vi "找球.vi"(1 "抬球电机继电器":T1, 2 "错误输入":errorcluster, 3 "光电门":T1, 4 "I/O":T11) -> (0 "错误输出":errorcluster)   [LabVIEW 2016]
uses:
  <vilib>/myRIO/Instrument Drivers/Onboard IO/PWM/typedefs/PWM Reference.ctl
  <vilib>/myRIO/Common/Instrument Driver Framework/Utilities/typedefs/myRIO Generic Hardware Reference.ctl
  <vilib>/myRIO/Common/Instrument Driver Framework/Utilities/typedefs/Hardware Version Enum.ctl
  <vilib>/myRIO/Common/Instrument Driver Framework/Utilities/typedefs/myRIO v1.0 Reference.ctl
  <vilib>/myRIO/Common/Instrument Driver Framework/Utilities/typedefs/Generic FPGA Reference.ctl
  <vilib>/myRIO/Common/Instrument Driver Framework/myRIO v1.0/PWM/typedefs/PWM Channels Enum.ctl
  <vilib>/myRIO/Instrument Drivers/Onboard IO/PWM/typedefs/PWM Configuration.ctl
  <vilib>/myRIO/Instrument Drivers/Onboard IO/DIO/typedefs/DIO Reference.ctl
  <vilib>/myRIO/Common/Instrument Driver Framework/myRIO v1.0/DIO/typedefs/DIO Channels List.ctl
  <vilib>/myRIO/Common/Instrument Driver Framework/myRIO v1.0/DIO/typedefs/DIO Channels Enum.ctl
  <vilib>/Utility/error.llb/Error Cluster From Error Code.vi
  <vilib>/myRIO/Common/Instrument Driver Framework/myRIO v1.0/DIO/vis/myRIO v1.0 Read DIO.vi
  <vilib>/myRIO/Common/Instrument Driver Framework/myRIO v1.0/DIO/vis/myRIO v1.0 Write DIO.vi
  <vilib>/myRIO/Instrument Drivers/Onboard IO/DIO/DIO.lvlib
  <vilib>/myRIO/Instrument Drivers/Onboard IO/PWM/PWM.lvlib
panel:
  out "error out":errorcluster
  out "拟合结果":T12
  out "速度":dbl[](array[numeric])
  out "前进一":bool
  out "前进二":bool
  out "旋转二":bool
  out "旋转一":bool
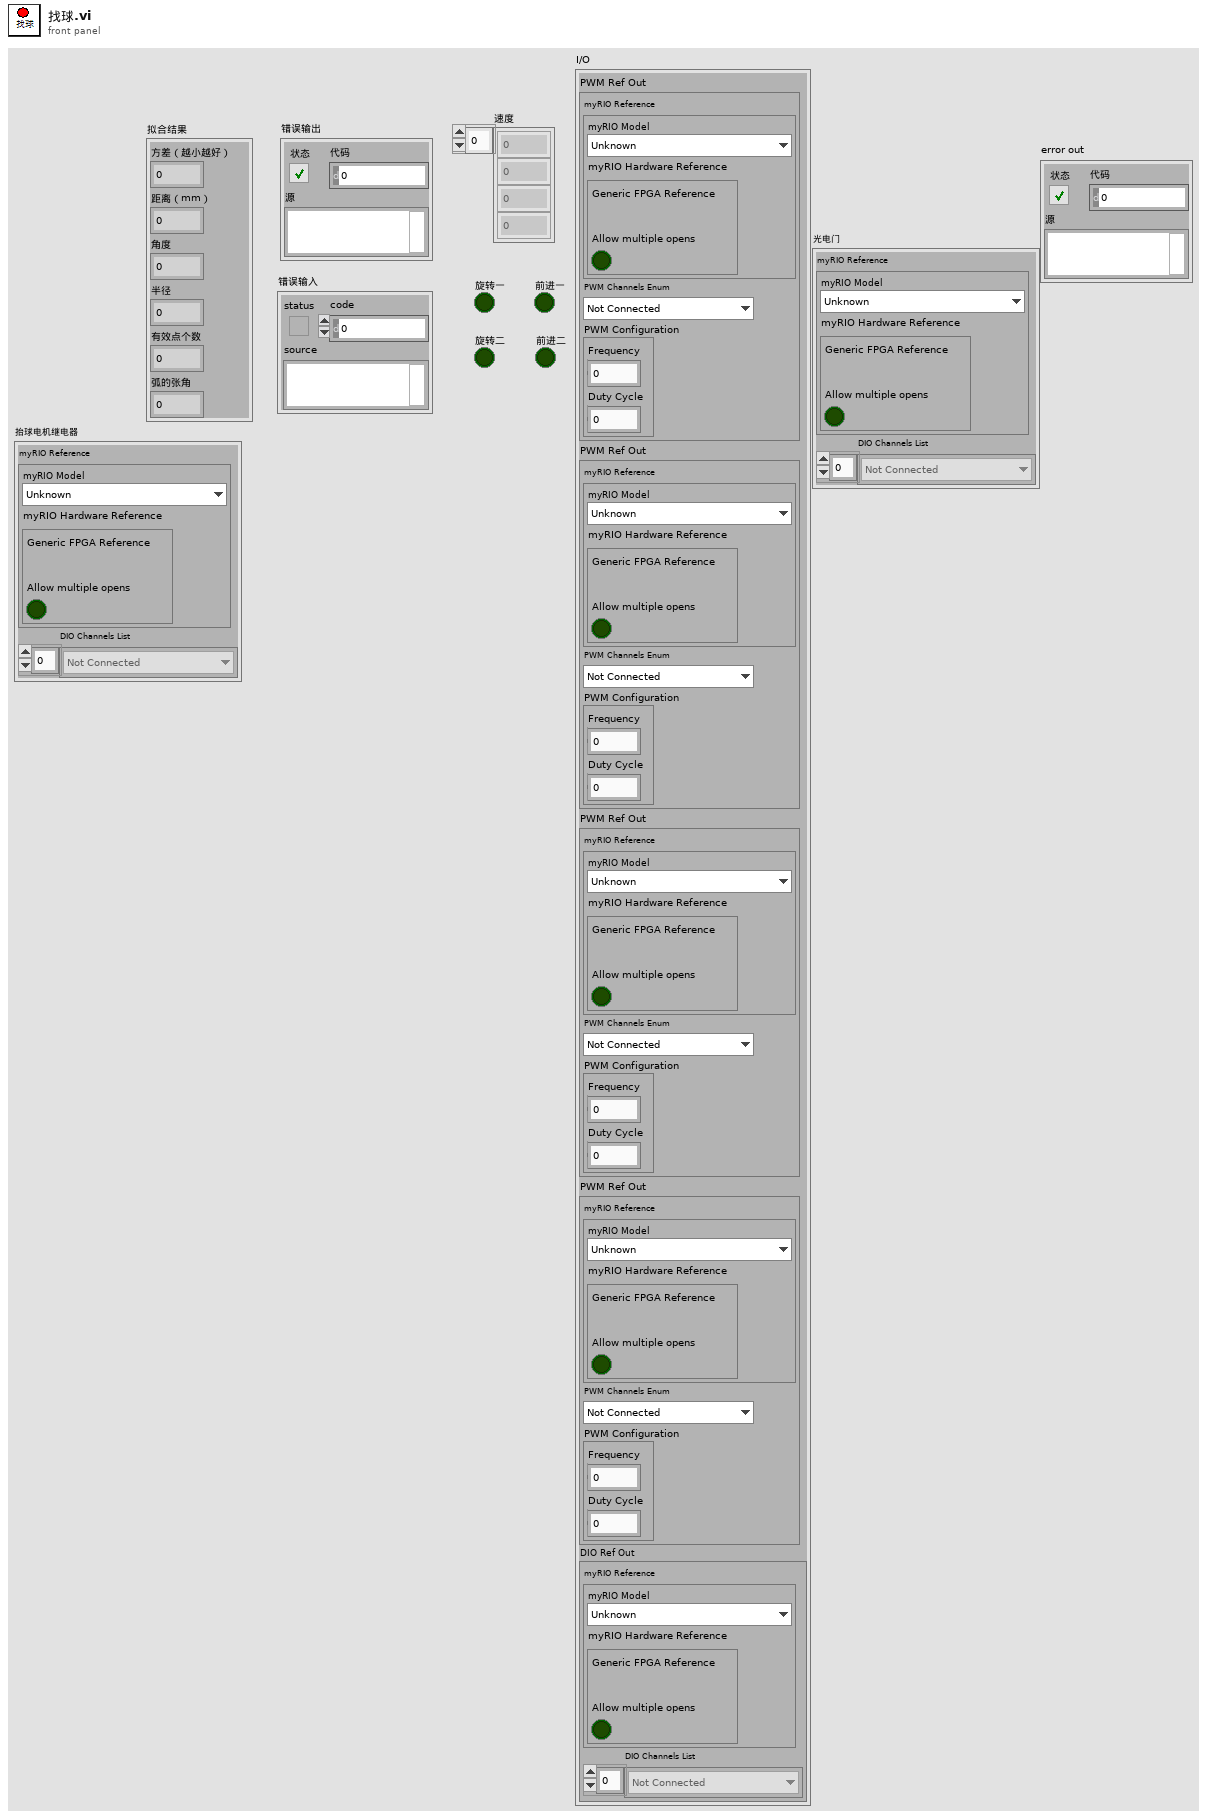
[diagram p1: front panel]
types:
  T1 = typedef "DIO.lvlib/DIO Reference.ctl" = cluster{"myRIO Reference":T2, "DIO Channels List":T6}
  T2 = typedef "myRIO Generic Hardware Reference.ctl" = cluster{"myRIO Model":T3, "myRIO Hardware Reference":T4}
  T3 = typedef "Hardware Version Enum.ctl" = enum16{"Unknown", "myRIO-1900", "myRIO-1950", "roboRIO", "NI ELVIS RIO CM"}
  T4 = typedef "myRIO v1.0 Reference.ctl" = cluster{"Generic FPGA Reference":T5, "Allow multiple opens":bool}
  T5 = typedef "Generic FPGA Reference.ctl" = refnum<k20>
  T6 = typedef "DIO Channels List.ctl" = T7[]
  T7 = typedef "DIO Channels Enum.ctl" = enum16{"Not Connected", "C/DIO0", "C/DIO1", "C/DIO2", "C/DIO3", "C/DIO4", "C/DIO5", "C/DIO6", "C/DIO7", "A/DIO0", "A/DIO1", "A/DIO2", "A/DIO3", "A/DIO4", "A/DIO5", "A/DIO6", "A/DIO7", "A/DIO8", "A/DIO9", "A/DIO10", "A/DIO11", "A/DIO12", "A/DIO13", "A/DIO14", "A/DIO15", "B/DIO0", "B/DIO1", "B/DIO2", "B/DIO3", "B/DIO4", "B/DIO5", "B/DIO6", "B/DIO7", "B/DIO8", "B/DIO9", "B/DIO10", "B/DIO11", "B/DIO12", "B/DIO13", "B/DIO14", "B/DIO15", "LED0", "LED1", "LED2", "LED3", "Button0", "DIO/DIO0", "DIO/DIO1", "DIO/DIO2", "DIO/DIO3", "DIO/DIO4", "DIO/DIO5", "DIO/DIO6", "DIO/DIO7", "DIO/DIO8", "DIO/DIO9", "SPI/CS0", "SPI/CS1", "SPI/CS2", "SPI/CS3", "LED RADIO (Green)", "LED RADIO (Red)", "LED COMM (Green)", "LED COMM (Red)", "LED MODE (Green)", "LED MODE (Red)"}
  T8 = typedef "PWM.lvlib/PWM Reference.ctl" = cluster{"myRIO Reference":T2, "PWM Channels Enum":T9, "PWM Configuration":T10}
  T9 = typedef "PWM Channels Enum.ctl" = enum16{"Not Connected", "C/PWM0", "C/PWM1", "A/PWM0", "A/PWM1", "A/PWM2", "B/PWM0", "B/PWM1", "B/PWM2", "PWM/PWM0", "PWM/PWM1", "PWM/PWM2", "PWM/PWM3", "PWM/PWM4", "PWM/PWM5", "PWM/PWM6", "PWM/PWM7", "PWM/PWM8", "PWM/PWM9"}
  T10 = typedef "PWM.lvlib/PWM Configuration.ctl" = cluster{"Frequency":dbl, "Duty Cycle":dbl}
  T11 = cluster{"PWM Ref Out":T8, "PWM Ref Out":T8, "PWM Ref Out":T8, "PWM Ref Out":T8, "DIO Ref Out":T1}
  T12 = cluster{"方差（越小越好）":dbl, "距离（mm）":dbl, "角度":dbl, "半径":dbl, "有效点个数":i32, "弧的张角":dbl}
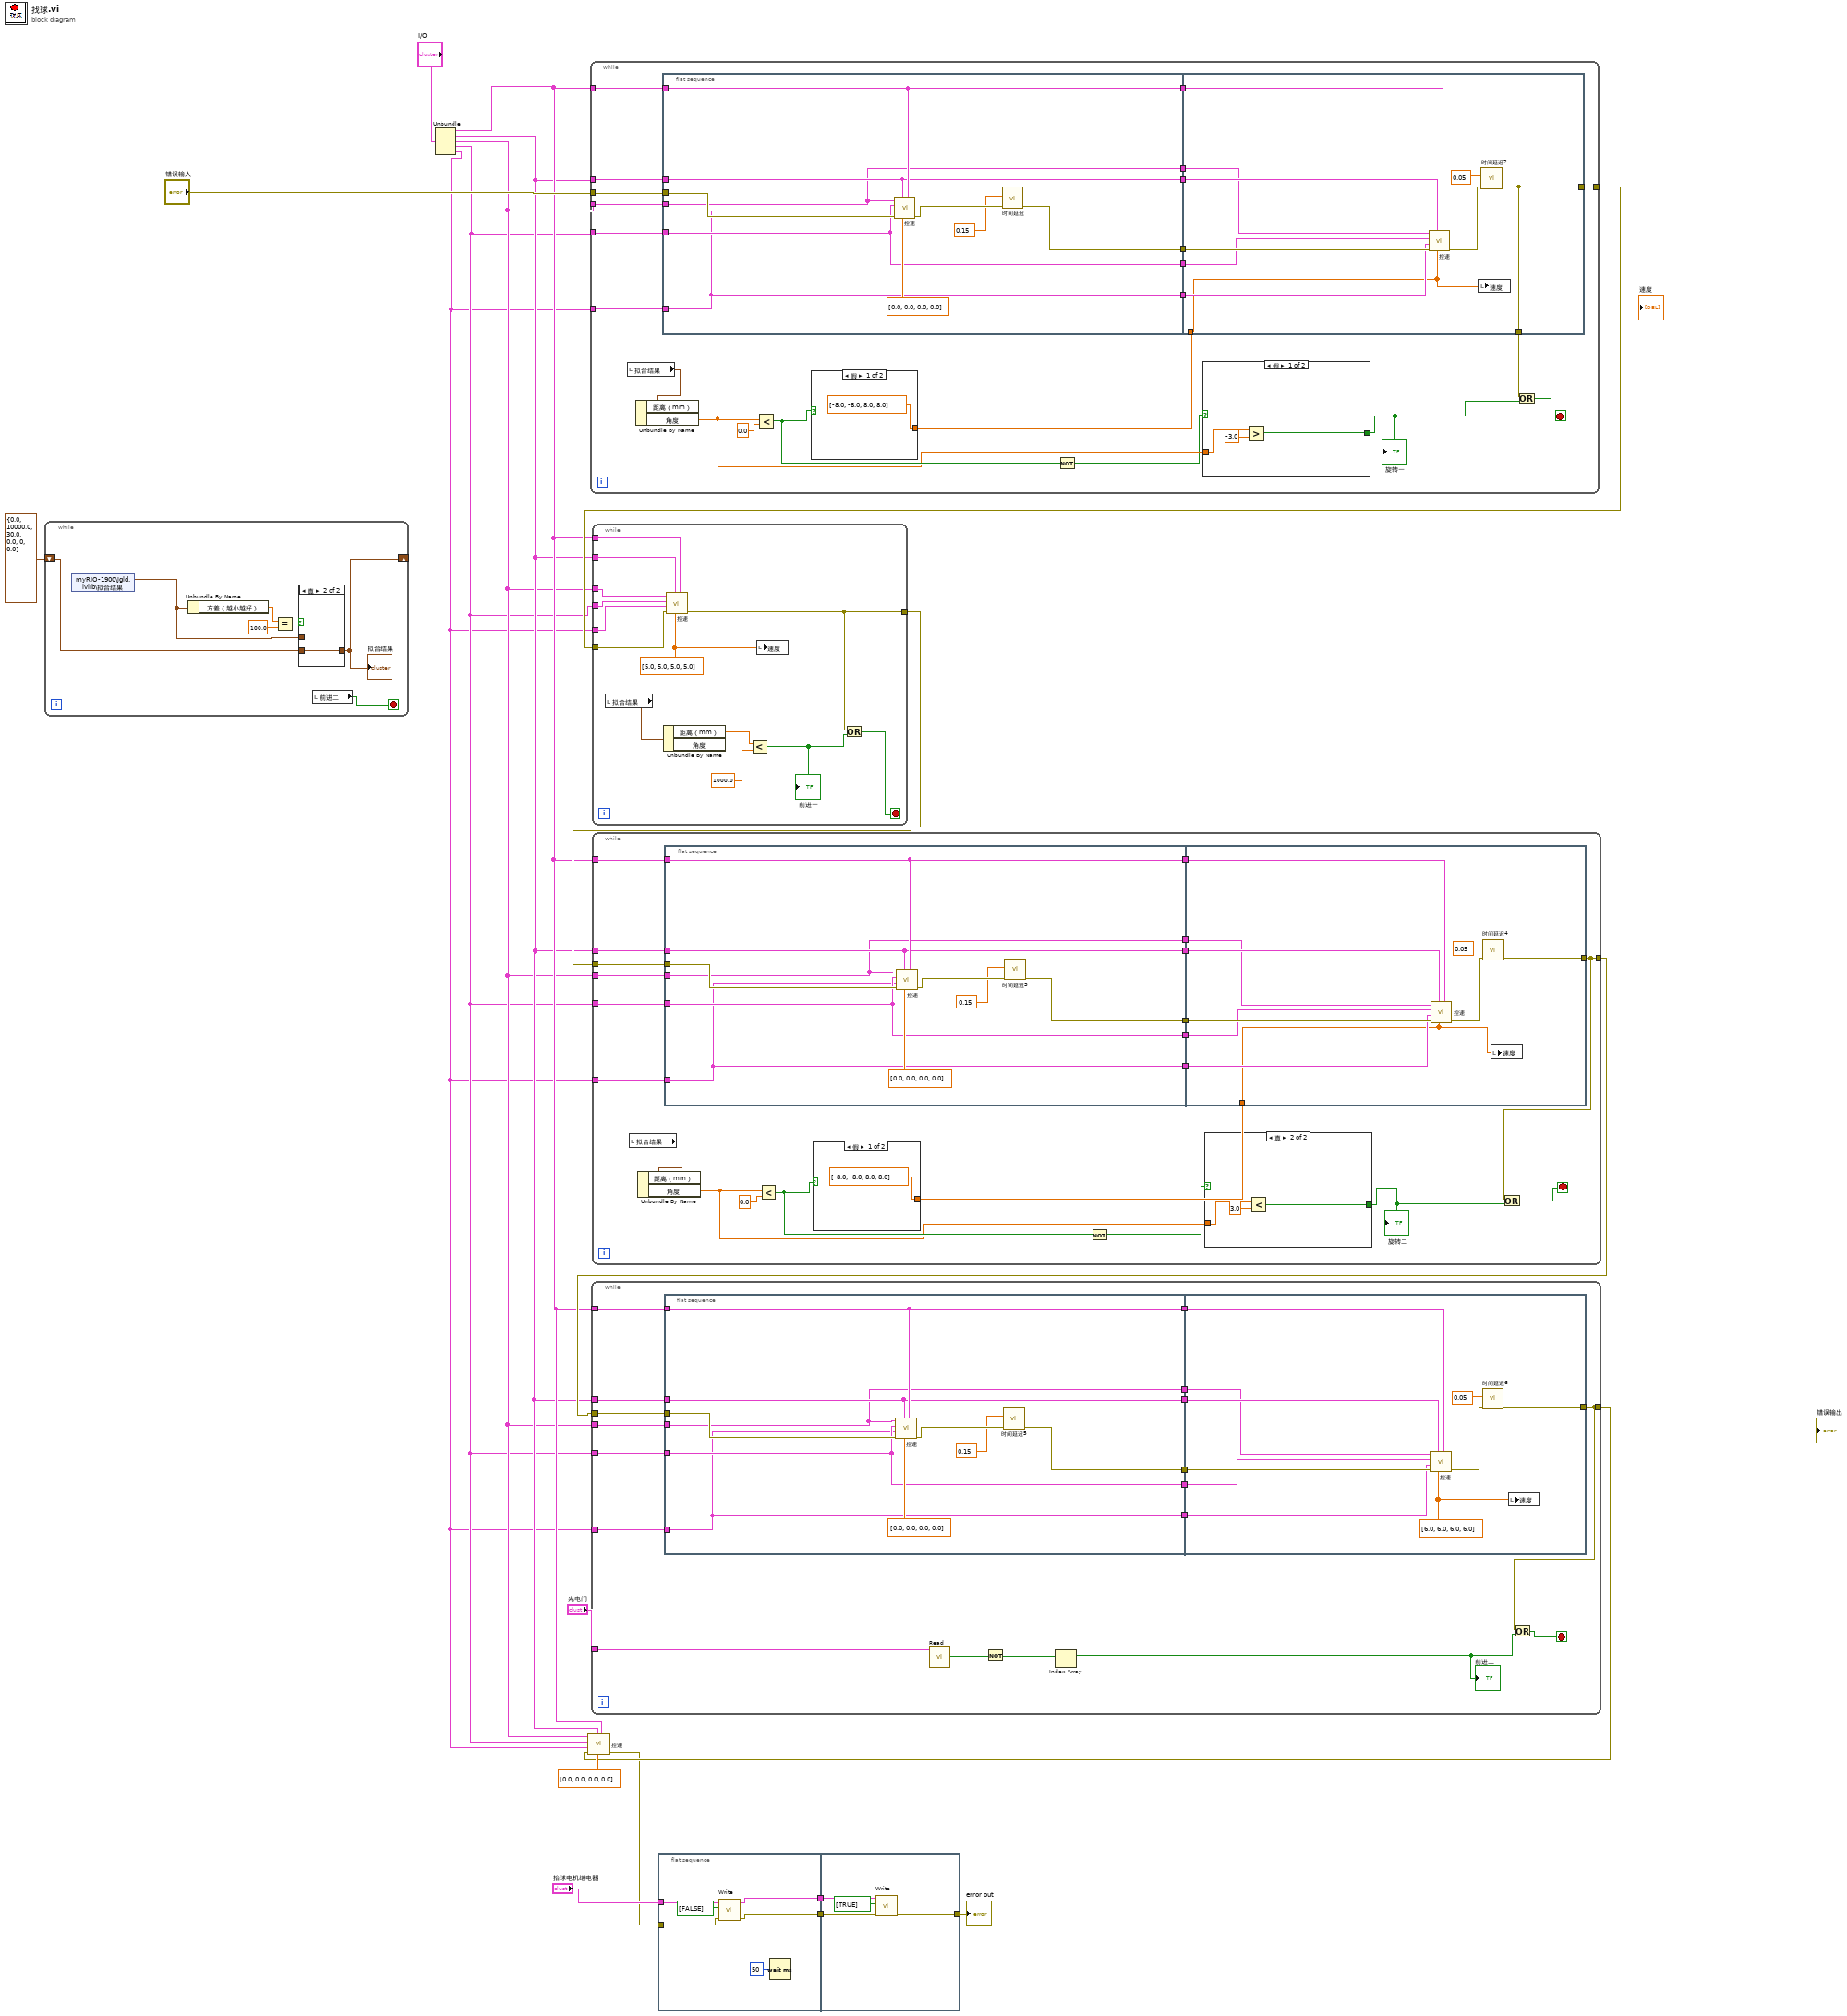
[diagram p0: block diagram]
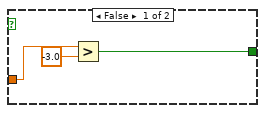
[diagram p3: hidden frame]
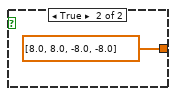
[diagram p4: hidden frame]
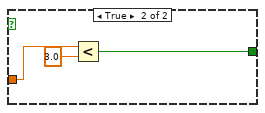
[diagram p5: hidden frame]
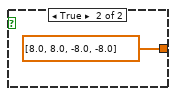
[diagram p6: hidden frame]
diagram:
  n1 = while {
    shift-right: [w22] -> _
    shift-left: T12 {"方差（越小越好）"=0.0, "距离（mm）"=10000.0, "角度"=30.0, "半径"=0.0, "有效点个数"=0, "弧的张角"=0.0} ("拟合结果") -> [w23]
    stop <- w21 stop-if-true
    n2 = shared-variable "myRIO-1900\\jgld.lvlib\\拟合结果"() -> (w20:T12)  [unwired: 1 in, 1 out]
    n3 = Unbundle By Name(w20) -> ("方差（越小越好）"=w26:dbl)
    n4 = Equal?(x=w26, y=100.0) -> (x = y?=w24:bool)
    n5 = case shown="真" w24 {
      tunnel: w23 -> [_ w28]
      tunnel: [w27 w28] -> w22
      tunnel: w20 -> [w27 _]
      frame False {
      }
      frame True {
      }
    }
    "拟合结果" <- w22
    n6 = local read "前进二"() -> (w21:bool)
  }
  n7 = Unbundle("I/O") -> ("PWM Ref Out"=w13:T8, "PWM Ref Out"=w12:T8, "PWM Ref Out"=w10:T8, "PWM Ref Out"=w9:T8, "DIO Ref Out"=w8:T1)
  n8 = while {
    tunnel: w13 -> [w46]
    tunnel: w12 -> [w45]
    tunnel: w9 -> [w44]
    tunnel: w10 -> [w43]
    tunnel: "错误输入" -> [w42]
    tunnel: w8 -> [w36]
    tunnel: [w33] -> w19
    stop <- w30 stop-if-true
    n9 = local read "拟合结果"() -> (w34:T12)
    n10 = Unbundle By Name(w34) -> ("角度"=w47:dbl)  [unwired: 1 out]
    n11 = flat-sequence {
      tunnel: w46 -> [w63]
      tunnel: w45 -> [w62]
      tunnel: w44 -> [w60]
      tunnel: w43 -> [w61]
      tunnel: w42 -> [w68]
      tunnel: [w64] -> w41
      tunnel: [w63] -> w40
      tunnel: [w62] -> w39
      tunnel: [w61] -> w38
      tunnel: [w60] -> w37
      tunnel: w36 -> [w59]
      tunnel: [w59] -> w35
      tunnel: w49 -> [w70]
      tunnel: w41 -> [w76]
      tunnel: w40 -> [w75]
      tunnel: w39 -> [w74]
      tunnel: w38 -> [w73]
      tunnel: w37 -> [w72]
      tunnel: w35 -> [w71]
      tunnel: [w69] -> w33
      tunnel: [w69] -> w31
      frame #0 {
        n12 = call "控速.vi"("PWM1"=w63, "速度"=dbl[] [0.0, 0.0, 0.0, 0.0], "PWM2"=w62, "错误输入（无错误）"=w68, "DIO"=w59, "PWM 4"=w60, "PWM 3"=w61) -> ("错误输出"=w66:errorcluster)  [unwired: 4 in]
        n13 = call "时间延迟"("error in (no error)"=w66, "Delay Time (s)"=0.15) -> ("error out"=w64:errorcluster)  [unwired: 9 in]
      }
      frame #1 {
        n14 = call "控速.vi"("PWM1"=w75, "速度"=w70, "PWM2"=w74, "错误输入（无错误）"=w76, "DIO"=w71, "PWM 4"=w72, "PWM 3"=w73) -> ("错误输出"=w78:errorcluster)  [unwired: 4 in]
        n15 = local write "速度"(w70) -> ()
        n16 = call "时间延迟2"("error in (no error)"=w78, "Delay Time (s)"=0.05) -> ("error out"=w69:errorcluster)  [unwired: 9 in]
      }
    }
    n17 = Less?(x=w47, y=0.0) -> (x < y?=w48:bool)
    n18 = case shown="假" w48 {
      tunnel: [dbl[] [-8.0, -8.0, 8.0, 8.0] ("速度") dbl[] [8.0, 8.0, -8.0, -8.0] ("速度")] -> w49
      frame False {
      }
      frame True {
      }
    }
    n19 = Not(x=w48) -> (.not. x?=w29:bool)
    n20 = case shown="假" w29 {
      tunnel: w47 -> [w53 w56]
      tunnel: [w51 w54] -> w32
      frame False {
        n21 = Greater?(x=w53, y=-3.0) -> (0:w51:bool)
      }
      frame True {
        n22 = Less?(x=w56, y=3.0) -> (x < y?=w54:bool)
      }
    }
    "旋转一" <- w32
    n23 = Or(x=w31, y=w32) -> (x .or. y?=w30:bool)
  }
  n24 = while {
    tunnel: w13 -> [w91]
    tunnel: w12 -> [w90]
    tunnel: w10 -> [w89]
    tunnel: w9 -> [w88]
    tunnel: w8 -> [w87]
    tunnel: w19 -> [w86]
    tunnel: [w80] -> w18
    stop <- w79 stop-if-true
    w82 = dbl[] [5.0, 5.0, 5.0, 5.0] ("速度")
    n25 = local read "拟合结果"() -> (w85:T12)
    n26 = Unbundle By Name(w85) -> ("距离（mm）"=w84:dbl)  [unwired: 1 out]
    n27 = call "控速.vi"("PWM1"=w91, "速度"=w82, "PWM2"=w90, "错误输入（无错误）"=w86, "DIO"=w87, "PWM 4"=w88, "PWM 3"=w89) -> ("错误输出"=w80:errorcluster)  [unwired: 4 in]
    n28 = Less?(x=w84, y=1000.0) -> (x < y?=w81:bool)
    "前进一" <- w81
    n29 = local write "速度"(w82) -> ()
    n30 = Or(x=w80, y=w81) -> (x .or. y?=w79:bool)
  }
  n31 = while {
    tunnel: w13 -> [w108]
    tunnel: w12 -> [w107]
    tunnel: w9 -> [w106]
    tunnel: w10 -> [w105]
    tunnel: w18 -> [w104]
    tunnel: w8 -> [w98]
    tunnel: [w94] -> w17
    stop <- w93 stop-if-true
    n32 = local read "拟合结果"() -> (w96:T12)
    n33 = Unbundle By Name(w96) -> ("角度"=w109:dbl)  [unwired: 1 out]
    n34 = flat-sequence {
      tunnel: w108 -> [w125]
      tunnel: w107 -> [w124]
      tunnel: w106 -> [w122]
      tunnel: w105 -> [w123]
      tunnel: w104 -> [w130]
      tunnel: [w126] -> w103
      tunnel: [w125] -> w102
      tunnel: [w124] -> w101
      tunnel: [w123] -> w100
      tunnel: [w122] -> w99
      tunnel: w98 -> [w121]
      tunnel: [w121] -> w97
      tunnel: w111 -> [w131]
      tunnel: w103 -> [w138]
      tunnel: w102 -> [w137]
      tunnel: w101 -> [w136]
      tunnel: w100 -> [w135]
      tunnel: w99 -> [w134]
      tunnel: w97 -> [w133]
      tunnel: [w132] -> w94
      frame #0 {
        n35 = call "控速.vi"("PWM1"=w125, "速度"=dbl[] [0.0, 0.0, 0.0, 0.0], "PWM2"=w124, "错误输入（无错误）"=w130, "DIO"=w121, "PWM 4"=w122, "PWM 3"=w123) -> ("错误输出"=w128:errorcluster)  [unwired: 4 in]
        n36 = call "时间延迟3"("error in (no error)"=w128, "Delay Time (s)"=0.15) -> ("error out"=w126:errorcluster)  [unwired: 9 in]
      }
      frame #1 {
        n37 = call "控速.vi"("PWM1"=w137, "速度"=w131, "PWM2"=w136, "错误输入（无错误）"=w138, "DIO"=w133, "PWM 4"=w134, "PWM 3"=w135) -> ("错误输出"=w140:errorcluster)  [unwired: 4 in]
        n38 = call "时间延迟4"("error in (no error)"=w140, "Delay Time (s)"=0.05) -> ("error out"=w132:errorcluster)  [unwired: 9 in]
        n39 = local write "速度"(w131) -> ()
      }
    }
    n40 = Less?(x=w109, y=0.0) -> (x < y?=w110:bool)
    n41 = case shown="假" w110 {
      tunnel: [dbl[] [-8.0, -8.0, 8.0, 8.0] ("速度") dbl[] [8.0, 8.0, -8.0, -8.0] ("速度")] -> w111
      frame False {
      }
      frame True {
      }
    }
    n42 = Not(x=w110) -> (.not. x?=w92:bool)
    n43 = case shown="真" w92 {
      tunnel: w109 -> [w115 w118]
      tunnel: [w113 w116] -> w95
      frame False {
        n44 = Greater?(x=w115, y=-3.0) -> (0:w113:bool)
      }
      frame True {
        n45 = Less?(x=w118, y=3.0) -> (x < y?=w116:bool)
      }
    }
    "旋转二" <- w95
    n46 = Or(x=w94, y=w95) -> (x .or. y?=w93:bool)
  }
  n47 = while {
    tunnel: w13 -> [w158]
    tunnel: w12 -> [w157]
    tunnel: w9 -> [w156]
    tunnel: w10 -> [w155]
    tunnel: w17 -> [w154]
    tunnel: w8 -> [w148]
    tunnel: [w146] -> w6
    tunnel: "光电门" -> [w141]
    stop <- w143 stop-if-true
    n48 = flat-sequence {
      tunnel: w158 -> [w163]
      tunnel: w157 -> [w162]
      tunnel: w156 -> [w160]
      tunnel: w155 -> [w161]
      tunnel: w154 -> [w168]
      tunnel: [w164] -> w153
      tunnel: [w163] -> w152
      tunnel: [w162] -> w151
      tunnel: [w161] -> w150
      tunnel: [w160] -> w149
      tunnel: w148 -> [w159]
      tunnel: [w159] -> w147
      tunnel: w153 -> [w176]
      tunnel: w152 -> [w175]
      tunnel: w151 -> [w174]
      tunnel: w150 -> [w173]
      tunnel: w149 -> [w172]
      tunnel: w147 -> [w171]
      tunnel: [w170] -> w146
      frame #0 {
        n49 = call "控速.vi"("PWM1"=w163, "速度"=dbl[] [0.0, 0.0, 0.0, 0.0], "PWM2"=w162, "错误输入（无错误）"=w168, "DIO"=w159, "PWM 4"=w160, "PWM 3"=w161) -> ("错误输出"=w166:errorcluster)  [unwired: 4 in]
        n50 = call "时间延迟5"("error in (no error)"=w166, "Delay Time (s)"=0.15) -> ("error out"=w164:errorcluster)  [unwired: 9 in]
      }
      frame #1 {
        w169 = dbl[] [6.0, 6.0, 6.0, 6.0] ("速度")
        n51 = call "控速.vi"("PWM1"=w175, "速度"=w169, "PWM2"=w174, "错误输入（无错误）"=w176, "DIO"=w171, "PWM 4"=w172, "PWM 3"=w173) -> ("错误输出"=w178:errorcluster)  [unwired: 4 in]
        n52 = call "时间延迟6"("error in (no error)"=w178, "Delay Time (s)"=0.05) -> ("error out"=w170:errorcluster)  [unwired: 9 in]
        n53 = local write "速度"(w169) -> ()
      }
    }
    n54 = call <vilib>:"Read.vi"("DIO Ref In"=w141) -> ("Values"=w145:bool[])  [unwired: 8 in, 2 out]
    n55 = Not(x=w145) -> (.not. x?=w144:bool[])
    n56 = Index Array(array=w144) -> (element=w142:bool)  [unwired: 1 in]
    "前进二" <- w142
    n57 = Or(x=w146, y=w142) -> (x .or. y?=w143:bool)
  }
  n58 = call "控速.vi"("PWM1"=w13, "速度"=dbl[] [0.0, 0.0, 0.0, 0.0], "PWM2"=w12, "错误输入（无错误）"=w6, "DIO"=w8, "PWM 4"=w9, "PWM 3"=w10) -> ("错误输出"=w2:errorcluster)  [unwired: 4 in]
  n59 = flat-sequence {
    tunnel: "抬球电机继电器" -> [w184]
    tunnel: [w181] -> w4
    tunnel: [w180] -> w3
    tunnel: w2 -> [w179]
    tunnel: w4 -> [w188]
    tunnel: w3 -> [w186]
    tunnel: [w185] -> w1
    frame #0 {
      n60 = call <vilib>:"Write.vi"("error in (no error)"=w179, "Values"=bool[] [FALSE], "DIO Ref In"=w184) -> ("error out"=w180:errorcluster, "DIO Ref Out"=w181:T1)  [unwired: 6 in]
      n61 = Wait (ms)(milliseconds to wait=u32 50 ("等待时间（毫秒）")) -> ()  [unwired: 1 out]
    }
    frame #1 {
      n62 = call <vilib>:"Write.vi"("error in (no error)"=w186, "Values"=bool[] [TRUE], "DIO Ref In"=w188) -> ("error out"=w185:errorcluster)  [unwired: 6 in, 1 out]
    }
  }
  "error out" <- w1
